vi "ReadCalFile.vi"(1 "Raw Spectrum":dbl[](array[numeric]), 2 "Wavelengths":dbl[](array[numeric])) -> (0 "Calibrated Spectrum":dbl[](array[numeric]))   [LabVIEW 2018]
panel:
  in  "New Cal File?":bool
  out "Wavelengths":waveform(dbl)[](array[waveform])=[{"t0"=timestamp(0 s since 1904-01-01), "dt"=0.0, "Y"=array[2028 elements], "attributes"=variant("datatype"=variant(string "DT_DOUBLE"), "description"=variant(string ""), "displaytype"=variant(string "Numeric"), "monotony"=variant(string "not calculated"), "novaluekey"=variant(string "not calculated"))}, {"t0"=timestamp(0 s since 1904-01-01), "dt"=0.0, "Y"=array[512 elements], "attributes"=variant("datatype"=variant(string "DT_DOUBLE"), "description"=variant(string ""), "displaytype"=variant(string "Numeric"), "monotony"=variant(string "not calculated"), "novaluekey"=variant(string "not calculated"))}]
  out "Calibrations":waveform(dbl)[](array[waveform])=[{"t0"=timestamp(0 s since 1904-01-01), "dt"=0.0, "Y"=array[2028 elements], "attributes"=variant("datatype"=variant(string "DT_DOUBLE"), "description"=variant(string "Input: [7]/Radiance_Vis (514), [6]/Vis_Subtracted (511)"), "displaytype"=variant(string "Numeric"), "maximum"=variant(dbl 517.9862907743333), "minimum"=variant(dbl -541.6497859037797), "monotony"=variant(string "not monotone"), "novaluekey"=variant(string "Yes"))}, {"t0"=timestamp(0 s since 1904-01-01), "dt"=0.0, "Y"=array[512 elements], "attributes"=variant("datatype"=variant(string "DT_DOUBLE"), "description"=variant(string "Input: [7]/Radiance_NIR (515), [6]/NIR_Subtracted (512)"), "displaytype"=variant(string "Numeric"), "maximum"=variant(dbl 0.8399345575398146), "minimum"=variant(dbl 0.005655809178791624), "monotony"=variant(string "not monotone"), "novaluekey"=variant(string "Yes"))}]
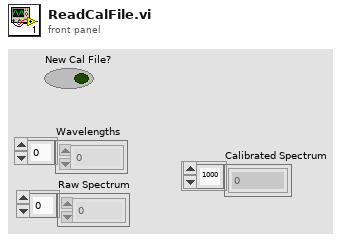
[diagram p1: front panel]
types:
  T1 = enum16{"open", "open or create", "create or replace", "create", "open (read-only)"}
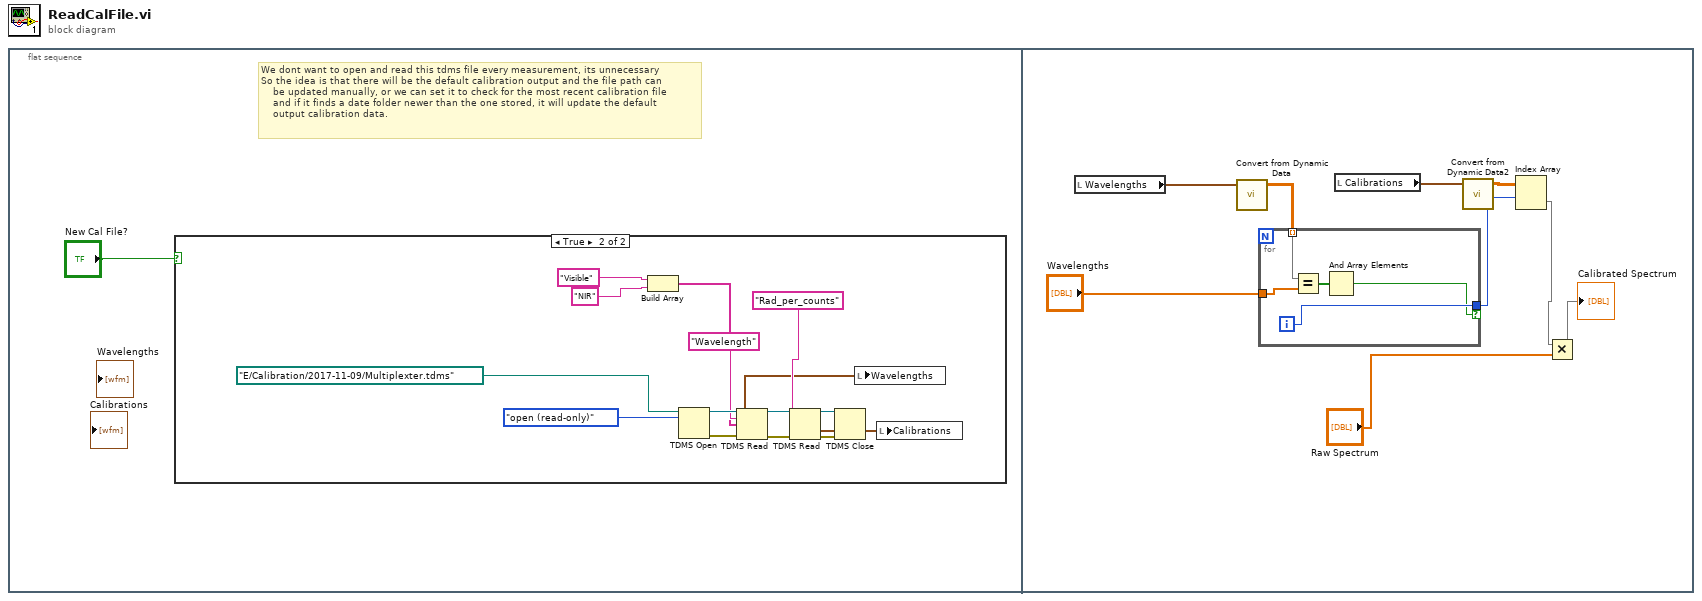
[diagram p0: block diagram]
diagram:
  n1 = flat-sequence {
    frame #0 {
      # "We dont want to open and read this tdms file every measurement, its unnecessary\nSo the idea is that there will be the default calibration output and the file path can \n    be updated manually, or we can set it to check for the most recent calibration file\n    and if it finds a date folder newer than the one stored, it will update the default \n    output calibration data."
      n2 = case shown="True" "New Cal File?" {
        frame False {
        }
        frame True {
          n3 = Build Array("Visible", "NIR") -> (w12:string[])
          n4 = TDMS Open(10:T1."open (read-only)" ("operation (0:open)"), 11:path "E:/Calibration/2017-11-09/Multiplexter.tdms" ("Normalization path")) -> (0:w14:errorcluster, 3:w15:refnum<k34>)  [unwired: 5 in]
          n5 = TDMS Read(0:w15, 5:"Wavelength" ("group name in"), 7:w12, 11:w14) -> (4:w11:refnum<k34>, 10:w2:waveform(dbl)[], 15:w10:errorcluster)  [unwired: 4 in, 3 out]
          n6 = TDMS Read(0:w11, 5:"Rad_per_counts", 11:w10) -> (4:w5:refnum<k34>, 10:w3:waveform(dbl)[], 15:w6:errorcluster)  [unwired: 5 in, 3 out]
          n7 = TDMS Close(8:w6, 11:w5) -> ()  [unwired: 2 out]
          n8 = local write "Wavelengths"(w2) -> ()
          n9 = local write "Calibrations"(w3) -> ()
        }
      }
    }
    frame #1 {
      n10 = local read "Wavelengths"() -> (w20:waveform(dbl)[])
      n11 = call "Convert from Dynamic Data"("Dynamic Data Type"=w20) -> ("Array"=w21:dbl[][])  [unwired: 3 in]
      n12 = for {
        tunnel: "Wavelengths" -> [w30]
        tunnel: [w28] -> w22 if=w27
        tunnel: w21 -> [w26] mode=indexing
        i -> [w28]
        n13 = Equal?(x=w26, y=w30) -> (x = y?=w29:bool[])
        n14 = And Array Elements(Boolean array=w29) -> (logical AND=w27:bool)
      }
      n15 = local read "Calibrations"() -> (w25:waveform(dbl)[])
      n16 = call "Convert from Dynamic Data2"("Dynamic Data Type"=w25) -> ("Array"=w24:dbl[][])  [unwired: 3 in]
      n17 = Index Array(array=w24, index (row)=w22) -> (element=w19:dbl[])  [unwired: 1 in]
      n18 = Multiply(x=w19, y="Raw Spectrum") -> (x*y=→"Calibrated Spectrum":dbl[])
    }
  }
